vi "Flush TDMS Log File.vi"(8 "error in (no error)":errorcluster, 11 "TDMS Log File in":refnum<class "TDMS Log File.lvclass">) -> (0 "error out":errorcluster, 3 "TDMS Log File out":refnum<class "TDMS Log File.lvclass">)   [LabVIEW 2015, in "TDMS Log File.lvclass"]
uses:
  TDMS Log File.lvclass
  TDMS Log File.lvclass/TDMS Log File.ctl
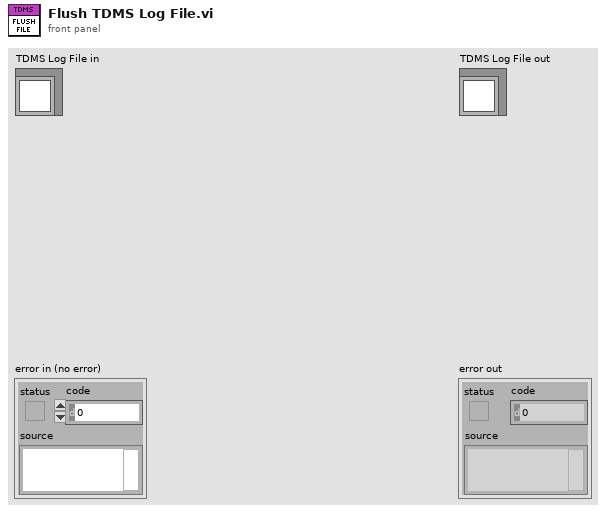
[diagram p1: front panel]
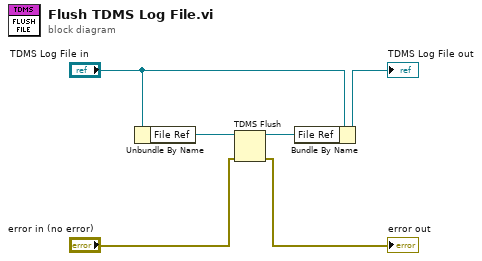
[diagram p0: block diagram]
diagram:
  n1 = Unbundle By Name("TDMS Log File in") -> ("File Ref"=w5:refnum<k34>)
  n2 = TDMS Flush(4:"error in (no error)", 7:w5) -> (0:→"error out":errorcluster, 3:w3:refnum<k34>)
  n3 = Bundle By Name(cluster="TDMS Log File in", "File Ref"=w3) -> (→"TDMS Log File out":refnum<class "TDMS Log File.lvclass">)
